vi "Set BrowerTree Model.vi"(8 "error in (no error)":errorcluster, 10 "BrowerTree.lvclass":refnum<class "BrowerTree.lvclass">, 11 "BrowerController in":refnum<class "BrowerController.lvclass">) -> (0 "error out":errorcluster, 3 "BrowerController out":refnum<class "BrowerController.lvclass">)   [LabVIEW 2015, in "BrowerController.lvclass"]
uses:
  BrowerController.lvclass
  Models/BrowerTree/BrowerTree.lvclass
  BrowerController.lvclass/BrowerController.ctl
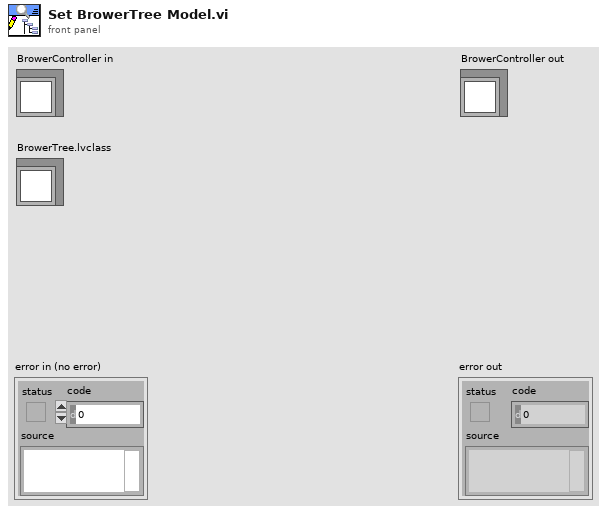
[diagram p1: front panel]
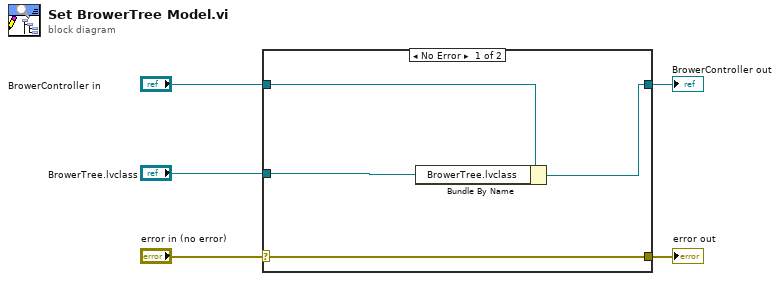
[diagram p0: block diagram]
diagram:
  n1 = case shown="No Error" "error in (no error)" {
    selector: "error in (no error)" -> [w9 w10]
    tunnel: [w9 w10] -> w4
    tunnel: [w7 w11] -> w2
    tunnel: "BrowerController in" -> [w8 w11]
    tunnel: "BrowerTree.lvclass" -> [w6 _]
    frame No Error {
      n2 = Bundle By Name(cluster=w8, "BrowerTree.lvclass"=w6) -> (w7:refnum<class "BrowerController.lvclass">)
    }
    frame Error {
    }
  }
  "error out" <- w4
  "BrowerController out" <- w2
